vi "Conveyer Belt MS Readings.vi"(1 "Conveyer Belt Information In":T1) -> (0 "Conveyer Belt Information Out":T1)   [LabVIEW 2012]
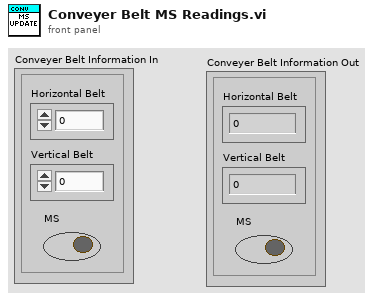
[diagram p1: front panel]
types:
  T1 = cluster{"Horizontal Belt":dbl, "Vertical Belt":dbl, "MS":bool}
  T2 = typedef "WPI_DigitalInputDevRef.ctl" = cluster{"DevStatus":errorcluster, "DIO Channel":T3, "Digital Module":T4}
  T3 = typedef "FPGA_DIOChannel.ctl" = enum8{"DIO 1", "DIO 2", "DIO 3", "DIO 4", "DIO 5", "DIO 6", "DIO 7", "DIO 8", "DIO 9", "DIO 10", "DIO 11", "DIO 12", "DIO 13", "DIO 14", "Invalid"}
  T4 = typedef "FPGA_TypedefDigitalModule.ctl" = enum16{"Digital Module 1", "Digital Module 2"}
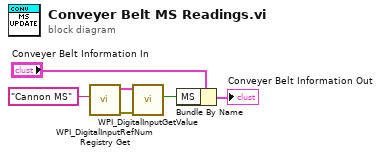
[diagram p0: block diagram]
diagram:
  n1 = call <vilib>:"WPI_DigitalInputRefNum Registry Get.vi"("refnum name"="Cannon MS") -> ("error out"=w6:errorcluster, "DigitalInputDevRef"=w5:T2)  [unwired: 9 in]
  n2 = call <vilib>:"WPI_DigitalInputGetValue.vi"("error in (no error)"=w6, "DigitalInputDevRef"=w5) -> ("Value"=w3:bool)  [unwired: 7 in, 2 out]
  n3 = Bundle By Name(cluster="Conveyer Belt Information In", "MS"=w3) -> (→"Conveyer Belt Information Out":T1)
